vi "load_from_file.vi"() -> ()   [LabVIEW 2023]
uses:
  <vilib>/addons/_office/excel.llb/Excel Get Data ([str]).vi
  <vilib>/Utility/NIReport.llb/NI_report.lvclass
  <vilib>/Utility/NIReport.llb/Excel/NI_Excel.lvclass
  <vilib>/addons/_office/NI_ReportGenerationToolkit.lvlib
panel:
  in  "?":bool
  in  "ACQUISITION FROM ARDUINO":bool
  in  "REQUEST TO SERVER":bool
  out "HUMIDITY TREND":dbl[](graph)
  out "PERCEIVED TEMP. TREND":dbl[](graph)
  out "TEMPERATURE TREND":dbl[](graph)
  in  "?":bool
  in  "file path":path
  # "LOAD DATA FROM .XLSX FILE"
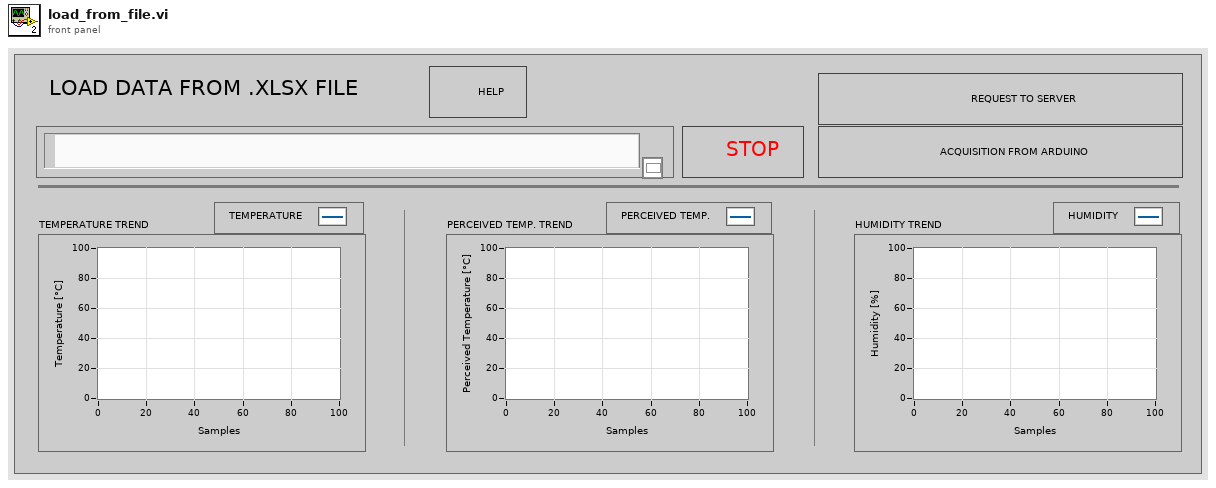
[diagram p1: front panel]
types:
  T1 = enum32{"Invalid", "Standard", "Closed", "Hidden", "Minimized", "Maximized"}
  T2 = enum16{"Standard Report", "HTML", "Word", "Excel"}
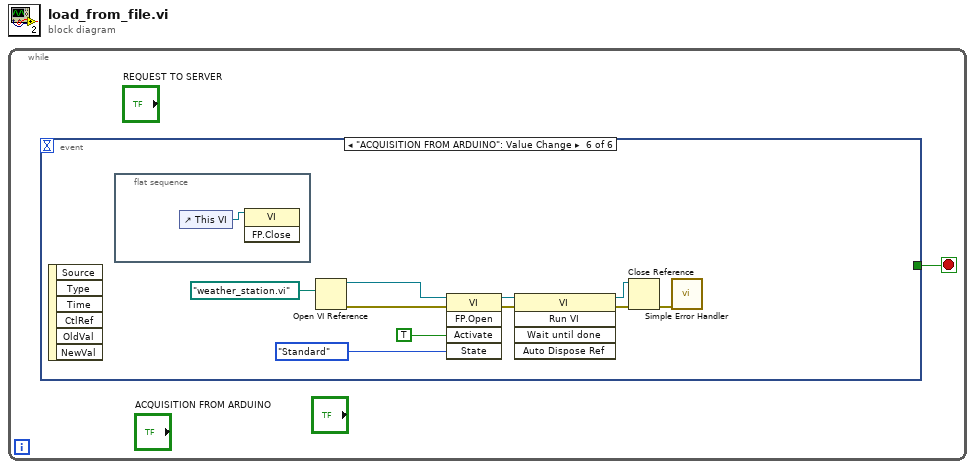
[diagram p0: block diagram]
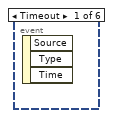
[diagram p2: hidden frame]
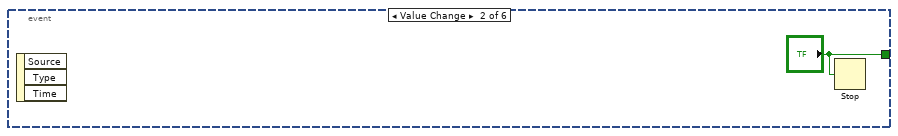
[diagram p3: hidden frame]
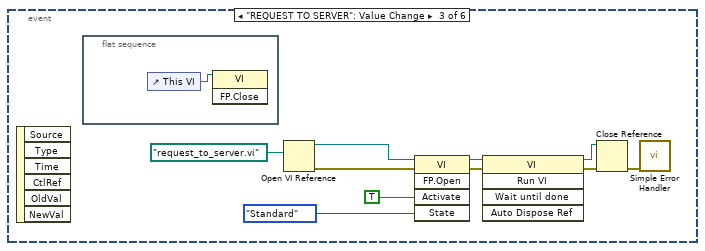
[diagram p4: hidden frame]
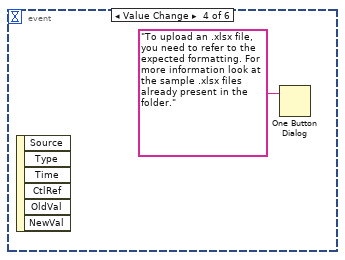
[diagram p5: hidden frame]
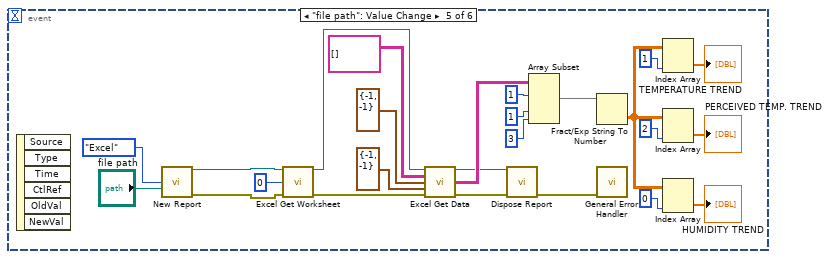
[diagram p6: hidden frame]
diagram:
  n1 = while {
    stop <- w1 stop-if-true
    n2 = event shown="[5] \"ACQUISITION FROM ARDUINO\": Value Change" {
      selector: _ -> [_ _ _ _ _ _]
      dyn-events: _ -> [_ _ _ _ _ _]
      timeout: _ -> [_ _ _ _ _ _]
      tunnel: [_ "?" _ _ _ _] -> w1
      event Timeout {
        n3 = event-data() -> ()  [unwired: 1 in, 3 out]
      }
      event Value Change {
        n4 = event-data() -> ()  [unwired: 1 in, 3 out]
        n5 = Stop(stop? (T)="?") -> ()
      }
      event "REQUEST TO SERVER": Value Change {
        n6 = event-data() -> ()  [unwired: 1 in, 6 out]
        n7 = flat-sequence {
          frame #0 {
            n8 = control-ref of="This VI"() -> (w13:refnum<vi>)
            n9 = invoke class="VI" method="FP.Close"(reference=w13) -> ()  [unwired: 2 in, 3 out]
          }
        }
        n10 = Open VI Reference(vi path=path "request_to_server.vi") -> (vi reference=w12:refnum<vi>, error out=w11:errorcluster)  [unwired: 5 in]
        n11 = invoke class="VI" method="FP.Open"(reference=w12, error in=w11, "Activate"=TRUE ("Activate?"), "State"=T1."Standard") -> (reference out=w3:refnum<vi>, error out=w8:errorcluster)  [unwired: 1 in, 3 out]
        n12 = invoke class="VI" method="Run VI"(reference=w3, error in=w8) -> (reference out=w6:refnum<vi>, error out=w7:errorcluster)  [unwired: 3 in, 3 out]
        n13 = Close Reference(reference=w6, error in (no error)=w7) -> (error out=w5:errorcluster)
        n14 = call <vilib>:"Simple Error Handler.vi"("error in (no error)"=w5) -> ()  [unwired: 4 in, 5 out]
      }
      event Value Change {
        n15 = event-data() -> ()  [unwired: 1 in, 6 out]
        n16 = One Button Dialog(message="To upload an .xlsx file, you need to refer to the expected formatting. For more information look at the sample .xlsx files already present in the folder.") -> ()  [unwired: 1 in, 1 out]
      }
      event "file path": Value Change {
        n17 = event-data() -> ()  [unwired: 1 in, 6 out]
        n18 = call <vilib>:"New Report.vi"("report type"=T2."Excel", "template (empty)"="file path") -> ("report out"=w28:refnum<class "NI_report.lvclass">, "error out"=w27:errorcluster)  [unwired: 4 in, 8 out]
        n19 = call <vilib>:"Excel Get Worksheet.vi"("report in"=w28, "worksheet index (0)"=0, "error in (no error)"=w27) -> ("report out"=w29:refnum<class "NI_report.lvclass">, "error out"=w30:errorcluster)  [unwired: 11 out]
        n20 = call-poly <vilib>:"Excel Get Data.vi"("report in"=w29, "data type"=string[][] [], "start (-1, -1)"=cluster{"row":i32, "column":i32} {"row"=-1, "column"=-1}, "end (-1, -1)"=cluster{"row":i32, "column":i32} {"row"=-1, "column"=-1}, "error in (no error)"=w30) -> ("report out"=w32:refnum<class "NI_report.lvclass">, "data"=w34:string[][], "error out"=w33:errorcluster)  [unwired: 8 out]
        n21 = call-dynamic "Dispose Report.vi"("report in"=w32, "error in (no error)"=w33) -> ("error out"=w31:errorcluster)  [unwired: 3 in, 10 out]
        n22 = Array Subset(array=w34, index (row)=1 ("index"), index (col)=1 ("index"), length (col)=3 ("length")) -> (w35:string[][])  [unwired: 1 in]
        n23 = Fract/Exp String To Number(string=w35) -> (number=w36:dbl[][])  [unwired: 3 in, 1 out]
        n24 = call <vilib>:"General Error Handler.vi"("error in (no error)"=w31) -> ()  [unwired: 3 in, 12 out]
        n25 = Index Array(array=w36, index (col)=1) -> (element=→"TEMPERATURE TREND":dbl[])  [unwired: 1 in]
        n26 = Index Array(array=w36, index (col)=2) -> (element=→"PERCEIVED TEMP. TREND":dbl[])  [unwired: 1 in]
        n27 = Index Array(array=w36, index (col)=0 ("disabled index (col)")) -> (element=→"HUMIDITY TREND":dbl[])  [unwired: 1 in]
      }
      event "ACQUISITION FROM ARDUINO": Value Change {
        n28 = event-data() -> ()  [unwired: 1 in, 6 out]
        n29 = flat-sequence {
          frame #0 {
            n30 = control-ref of="This VI"() -> (w50:refnum<vi>)
            n31 = invoke class="VI" method="FP.Close"(reference=w50) -> ()  [unwired: 2 in, 3 out]
          }
        }
        n32 = Open VI Reference(vi path=path "weather_station.vi") -> (vi reference=w49:refnum<vi>, error out=w48:errorcluster)  [unwired: 5 in]
        n33 = invoke class="VI" method="FP.Open"(reference=w49, error in=w48, "Activate"=TRUE ("Activate?"), "State"=T1."Standard") -> (reference out=w45:refnum<vi>, error out=w44:errorcluster)  [unwired: 1 in, 3 out]
        n34 = invoke class="VI" method="Run VI"(reference=w45, error in=w44) -> (reference out=w42:refnum<vi>, error out=w43:errorcluster)  [unwired: 3 in, 3 out]
        n35 = Close Reference(reference=w42, error in (no error)=w43) -> (error out=w41:errorcluster)
        n36 = call <vilib>:"Simple Error Handler.vi"("error in (no error)"=w41) -> ()  [unwired: 4 in, 5 out]
      }
    }
  }
